vi "DriveDistanceXAdvanced.vi"(2 "Parameter String":string, 3 "Reinit":bool) -> (0 "Error Out":errorcluster, 1 "Increment":bool)   [LabVIEW 2020]
doc: "The swerve drive base will translate in the field-centric X direction at a speed specified by the joystick command. This is a \"medium smart\" algorithm, there is an orientation lock and overshoot prevention. Any complex or critical translations should be handled using either the Path Follower or auto-targeting. \n\nParameters:\n1. relative travel distance in the field-centric X direction --> (in) [-630,630]\n2. undershoot error- the number of inches under the goal allowed --> (in) [0,630]\n3. overshoot error- the number of inches over the goal allowed --> (in) [0,630]\n4. timeout -->(ms) -1 to ignore [-1,15000]"
uses:
  SafeParser_Float.vi
  SafeParser_Integer.vi
  drivercommands.vi
  sensordata.vi
panel:
  out "Rotation PID":T1(graph)
  in  "PID Tuning Rotation":T2={"Kp"=0.007, "Ki"=0.03, "Kd"=0.001, "N-Diff"=5, "N-Int"=10, "Int Error Window"=30.0, "Max Ouput"=1.0, "Min Output"=-1.0} {"Int Error Window" min=0.0; "N-Int" min=2; "N-Diff" min=2; "Kd" min=0.0; "Ki" min=0.0; "Kp" min=0.0}
  in  "Time in Range (ms)":u32=1000
  out "Drive PID":T1(graph)
  in  "Plots?":bool
  in  "PID Tuning Drive":T2={"Kp"=0.01, "Ki"=0.0, "Kd"=0.0, "N-Diff"=10, "N-Int"=20, "Int Error Window"=0.5, "Max Ouput"=1.0, "Min Output"=-1.0} {"Int Error Window" min=0.0; "N-Int" min=2; "N-Diff" min=2; "Kd" min=0.0; "Ki" min=0.0; "Kp" min=0.0}
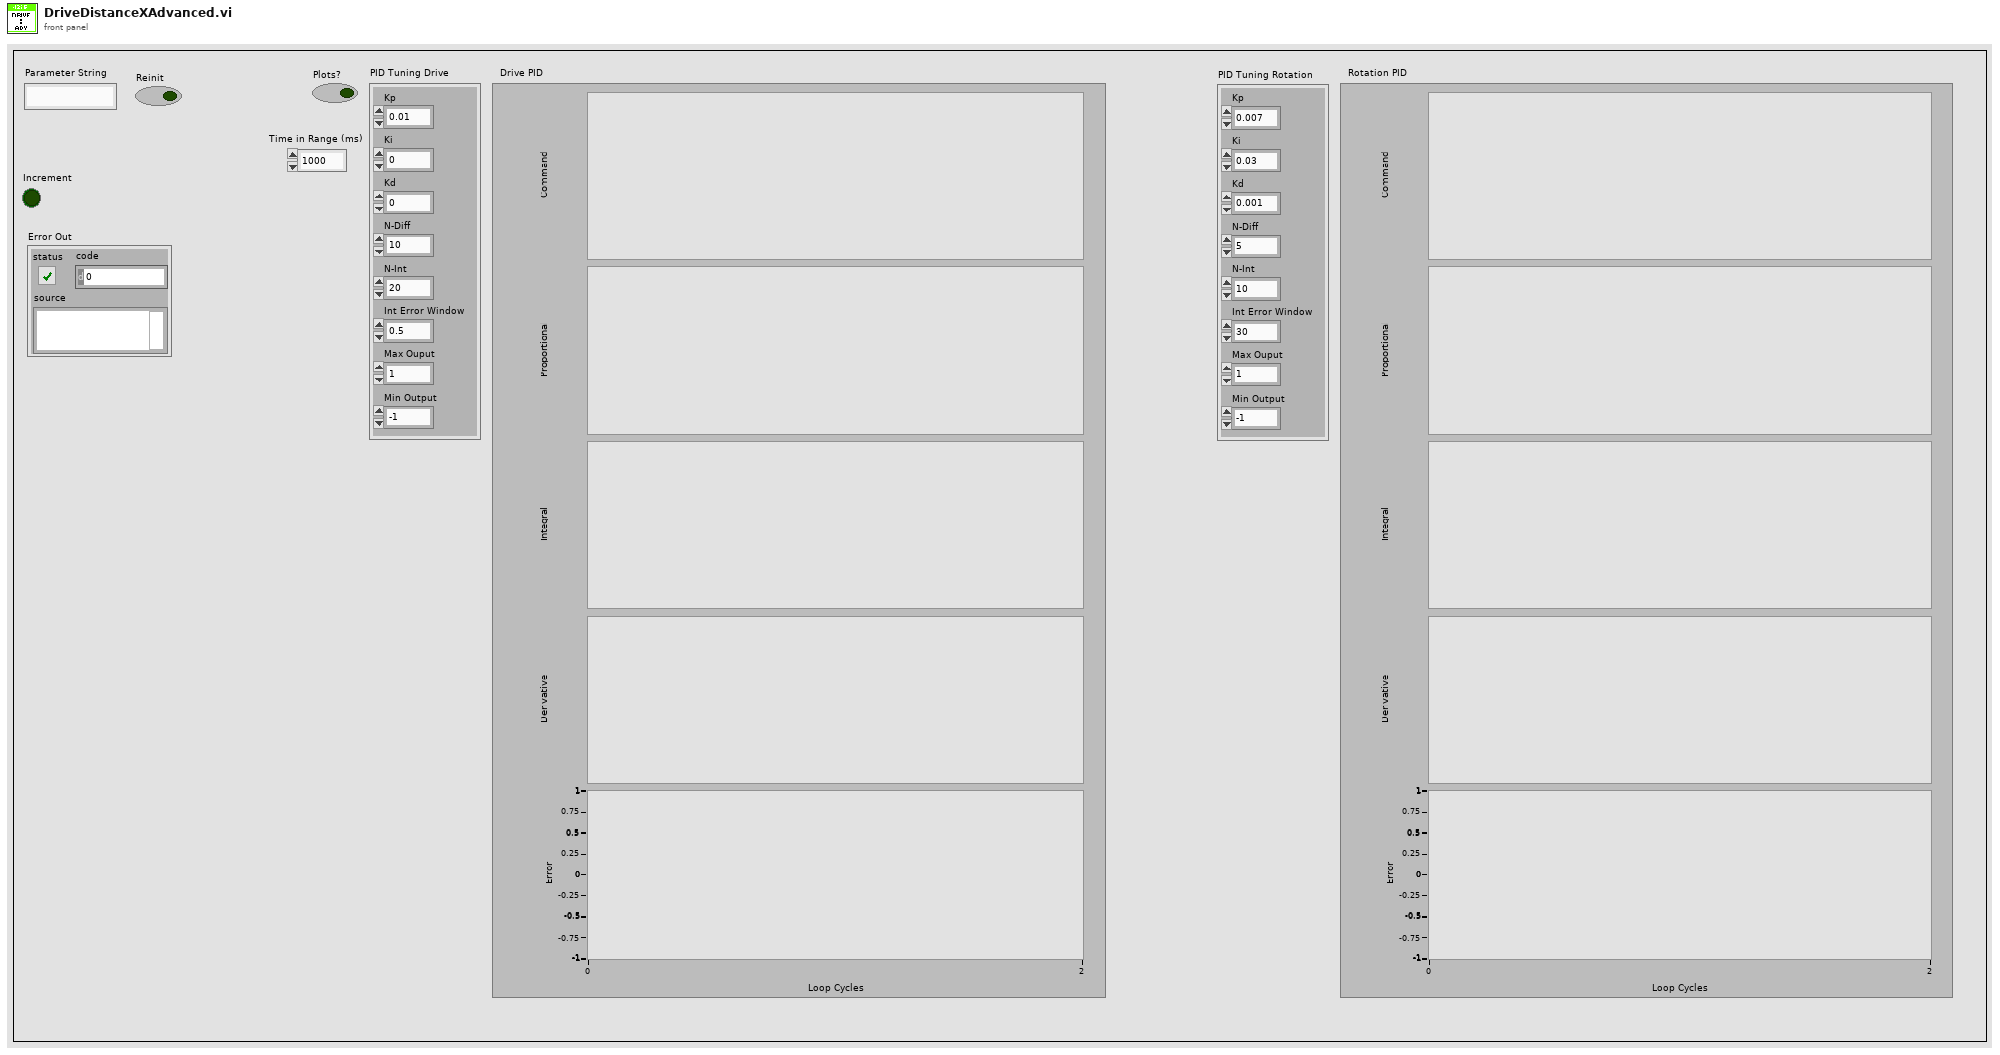
[diagram p1: front panel]
types:
  T1 = cluster{"Command":dbl, "Proportional":dbl, "Integral":dbl, "Derivative":dbl, "Goal":dbl}
  T2 = cluster{"Kp":dbl, "Ki":dbl, "Kd":dbl, "N-Diff":i32, "N-Int":i32, "Int Error Window":dbl, "Max Ouput":dbl, "Min Output":dbl}
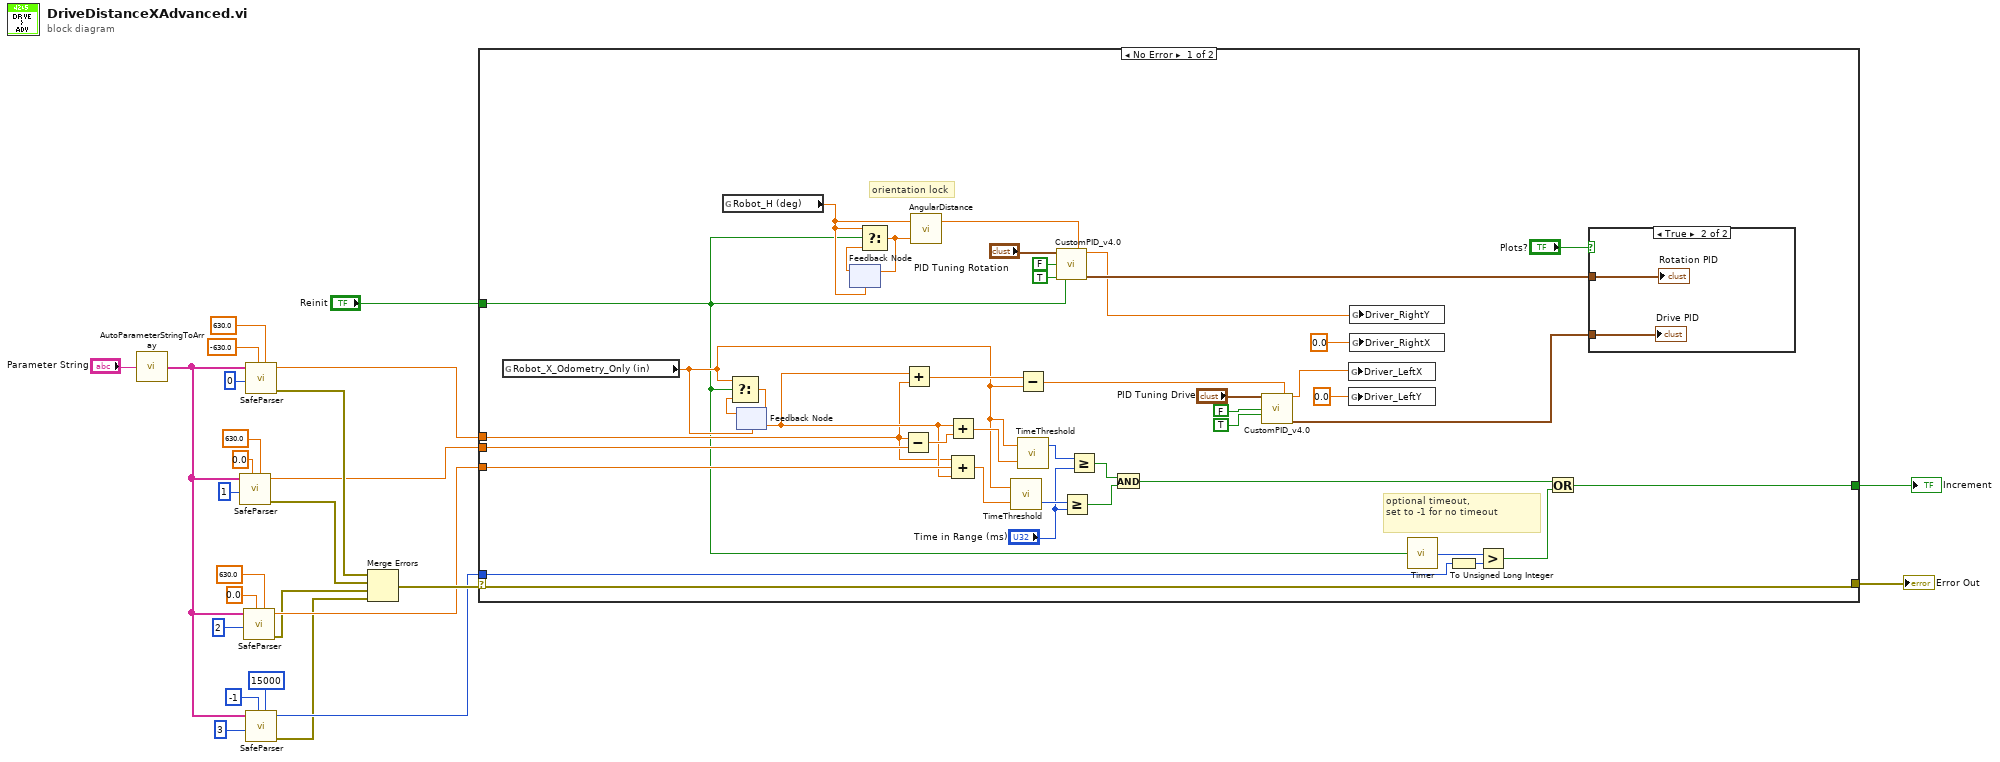
[diagram p0: block diagram]
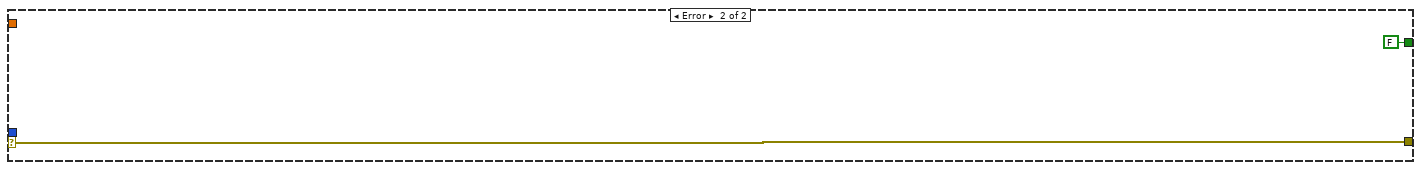
[diagram p3: hidden frame]
diagram:
  n1 = call "AutoParameterStringToArray.vi"("Parameter String"="Parameter String") -> ("Parsed Parameters"=w5:string[])
  n2 = call-poly "SafeParser.vi"("Maximum"=630.0, "Minimum"=0.0, "Array Index"=1 ("Parameter Index"), "String Array"=w5) -> ("Error Out"=w19:errorcluster, "Typecast  Value"=w16:dbl)  [unwired: 6 in]
  n3 = call-poly "SafeParser.vi"("Maximum"=630.0, "Minimum"=0.0, "Array Index"=2 ("Parameter Index"), "String Array"=w5) -> ("Error Out"=w9:errorcluster, "Typecast  Value"=w10:dbl)  [unwired: 6 in]
  n4 = call-poly "SafeParser.vi"("Maximum"=630.0, "Minimum"=-630.0, "Array Index"=0 ("Parameter Index"), "String Array"=w5) -> ("Error Out"=w18:errorcluster, "Typecast  Value"=w8:dbl)  [unwired: 6 in]
  n5 = call-poly "SafeParser.vi"("Maximum"=15000, "Minimum"=-1, "Array Index"=3 ("Parameter Index"), "String Array"=w5) -> ("Error Out"=w2:errorcluster, "Typecast  Value"=w3:i32)  [unwired: 6 in]
  n6 = Merge Errors(w18, w19, w9, w2) -> (w17:errorcluster)
  n7 = case shown="No Error" w17 {
    selector: w17 -> [w66 w71]
    tunnel: [w29 FALSE] -> w1
    tunnel: "Reinit" -> [w33 _]
    tunnel: [w66 w71] -> w25
    tunnel: w8 -> [w57 _]
    tunnel: w16 -> [w61 _]
    tunnel: w10 -> [w62 _]
    tunnel: w3 -> [w32 _]
    frame No Error {
      # "optional timeout,\nset to -1 for no timeout"
      # "orientation lock"
      n8 = global read "sensordata.vi" "Robot_X_Odometry_Only (in)"() -> (w46:dbl)
      n9 = global read "sensordata.vi" "Robot_H (deg)"() -> (w44:dbl)
      n10 = feedback #1(w46) -> (w60:dbl)
      n11 = Select(t=w46, s=w33, f=w60) -> (s? t:f=w58:dbl)
      n12 = feedback-in #1(w58) -> ()
      n13 = feedback #2(w44) -> (w42:dbl)
      n14 = Select(t=w44, s=w33, f=w42) -> (s? t:f=w43:dbl)
      n15 = feedback-in #2(w43) -> ()
      n16 = Subtract(x=w57, y=w61) -> (x-y=w59:dbl)
      n17 = Add(x=w58, y=w57) -> (x+y=w56:dbl)
      n18 = call "AngularDistance.vi"("Goal Angle (deg) [0,360]"=w43, "Current Angle (deg) [-Inf,+Inf]"=w44) -> ("Signed Angular Distance (deg) [-180,+180]"=w36:dbl)  [unwired: 1 out]
      n19 = Add(x=w58, y=w59) -> (x+y=w50:dbl)
      n20 = Compound Arithmetic op=ADD(w57, w62, w58) -> (w53:dbl)
      n21 = call "TimeThreshold.vi"("Threshold"=w53, "Current Value"=w46) -> ("Time Below Threshold (ms)"=w52:u32)  [unwired: 1 out]
      n22 = Subtract(x=w56, y=w46) -> (x-y=w45:dbl)
      n23 = call "TimeThreshold.vi"("Threshold"=w50, "Current Value"=w46) -> ("Time Above Threshold (ms)"=w49:u32)  [unwired: 1 out]
      n24 = call "CustomPID_v4.0.vi"("PID Tuning Parameters"="PID Tuning Rotation", "Custom Error Calculation"=w36, "Reset on Goal Change ?"=FALSE, "Use Custom Error Calculation ?"=TRUE, "Reinit"=w33) -> ("Command"=w37:dbl, "Controller Summary"=w38:T1)  [unwired: 7 in, 2 out]
      n25 = Greater Or Equal?(x=w52, y="Time in Range (ms)") -> (x >= y?=w51:bool)
      n26 = Greater Or Equal?(x=w49, y="Time in Range (ms)") -> (x >= y?=w47:bool)
      n27 = And(x=w47, y=w51) -> (x .and. y?=w31:bool)
      n28 = call "CustomPID_v4.0.vi"("PID Tuning Parameters"="PID Tuning Drive", "Custom Error Calculation"=w45, "Reset on Goal Change ?"=FALSE, "Use Custom Error Calculation ?"=TRUE) -> ("Command"=w28:dbl, "Controller Summary"=w54:T1)  [unwired: 8 in, 2 out]
      n29 = global write "drivercommands.vi" "Driver_LeftX"(w28) -> ()
      n30 = global write "drivercommands.vi" "Driver_LeftY"(0.0 ("Driver_LeftY")) -> ()
      n31 = global write "drivercommands.vi" "Driver_RightY"(w37) -> ()
      n32 = global write "drivercommands.vi" "Driver_RightX"(0.0 ("Driver_RightX")) -> ()
      n33 = call "Timer.vi"("Reset Timer"=w33) -> ("Time (ms)"=w34:u32)
      n34 = To Unsigned Long Integer(number=w32) -> (unsigned 32bit integer=w35:u32)
      n35 = Greater?(x=w34, y=w35) -> (0:w30:bool)
      n36 = Or(x=w31, y=w30) -> (x .or. y?=w29:bool)
      n37 = case shown="True" "Plots?" {
        tunnel: w54 -> [_ w69]
        tunnel: w38 -> [_ w68]
        frame False {
        }
        frame True {
          "Drive PID" <- w69
          "Rotation PID" <- w68
        }
      }
    }
    frame Error {
    }
  }
  "Increment" <- w1
  "Error Out" <- w25
